vi "MaxMinAvg.vi"(0 "Measurement":fxp<+/-,24,5>, 1 "Index":i32) -> (2 "Minimum Value":fxp<+/-,24,4> format="%.14f", 3 "Maximum Value":fxp<+/-,24,4> format="%.14f", 4 "Average Value":sgl)   [LabVIEW 2018]
panel:
  # "Calculate min, max\nand average values.\n\nIf index is 0, it is assumed \nthe first input is received and\nmin, max and averages will be\nset to this value.\n\nOtherwise, it is asusmed next value is received.\nCurrent Min, Max  values are compared with the\nnew value and new average is calculated."
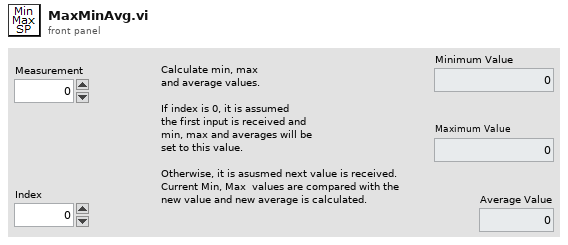
[diagram p1: front panel]
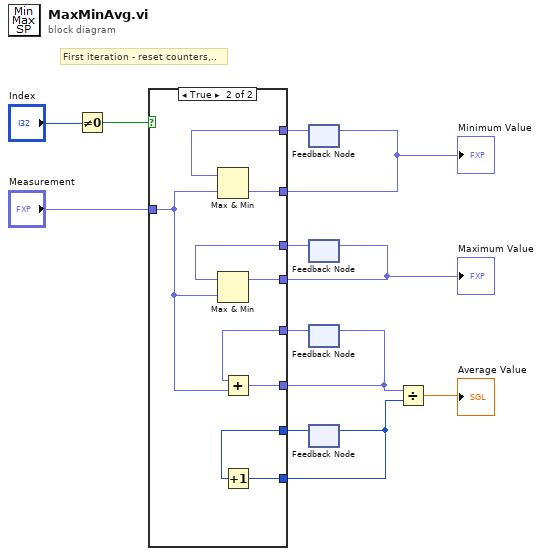
[diagram p0: block diagram]
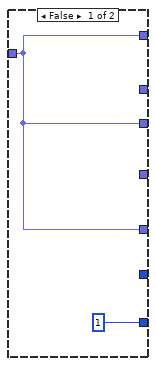
[diagram p2: hidden frame]
diagram:
  # "First iteration - reset counters,.."
  n1 = Not Equal To 0?(x="Index") -> (x != 0?=w10:bool)
  n2 = feedback #1() -> (w12:fxp<+/-,24,5>)  [unwired: 1 in]
  n3 = feedback #2() -> (w9:fxp<+/-,24,5>)  [unwired: 1 in]
  n4 = feedback #3() -> (w4:fxp<+/-,35,16>)  [unwired: 1 in]
  n5 = feedback #4() -> (w5:i32)  [unwired: 1 in]
  n6 = case shown="True" w10 {
    tunnel: "Measurement" -> [w13 w19]
    tunnel: w12 -> [_ w20]
    tunnel: w9 -> [_ w18]
    tunnel: [1 w23] -> w7
    tunnel: [w13 w17] -> w8
    tunnel: w5 -> [_ w22]
    tunnel: w4 -> [_ w21]
    tunnel: [w13 w16] -> w1
    tunnel: [w13 w15] -> w2
    frame False {
    }
    frame True {
      n7 = Max & Min(x=w20, y=w19) -> (min(x,y)=w15:fxp<+/-,24,5>)  [unwired: 1 out]
      n8 = Max & Min(x=w18, y=w19) -> (max(x,y)=w16:fxp<+/-,24,5>)  [unwired: 1 out]
      n9 = Add(x=w21, y=w19) -> (x+y=w17:fxp<+/-,32,16>)
      n10 = Increment(x=w22) -> (x+1=w23:i32)
    }
  }
  "Maximum Value" <- w1
  "Minimum Value" <- w2
  n11 = feedback-in #1(w2) -> ()
  n12 = feedback-in #2(w1) -> ()
  n13 = feedback-in #3(w8) -> ()
  n14 = feedback-in #4(w7) -> ()
  n15 = Divide(x=w8, y=w7) -> (x/y=→"Average Value":sgl)
